vi "Auto_Routine_QuickAuto.vi"(8 "error in (no error)":errorcluster, 9 "Distance(Back)":dbl, 10 "Game Piece":T1, 11 "Position":T2=enum."Middle") -> (0 "error out":errorcluster)   [LabVIEW 2023]
uses:
  Arm/ArmPositionPreset.ctl
  Arm/ArmGamePiecePreset.ctl
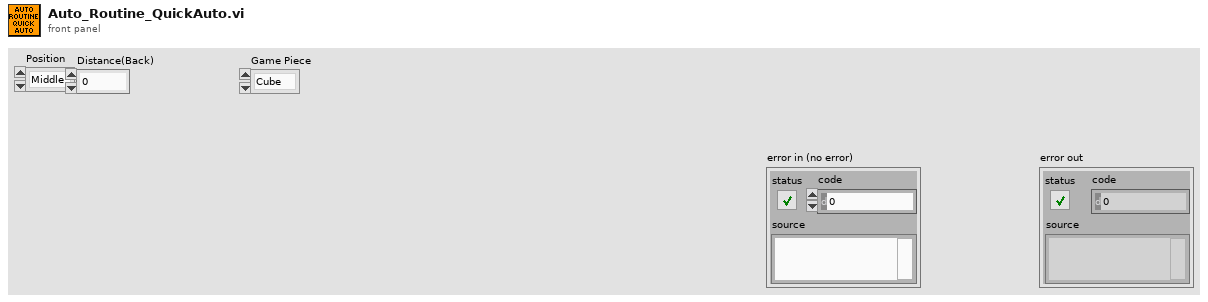
[diagram p1: front panel]
types:
  T1 = typedef "ArmGamePiecePreset.ctl" = enum16{"Cube", "Cone"}
  T2 = typedef "ArmPositionPreset.ctl" = enum16{"Upper", "Lower", "Middle", "Home", "Shelf", "Floor", "HalfFloor", "HalfHome"}
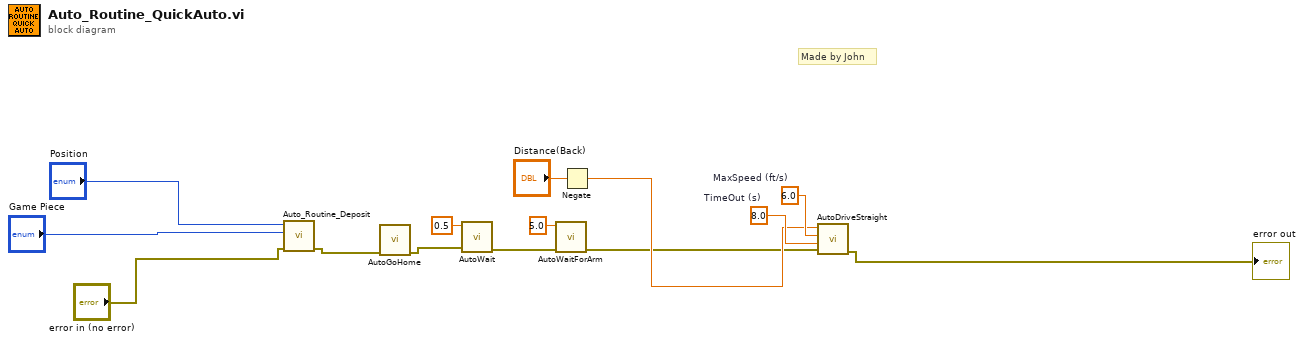
[diagram p0: block diagram]
diagram:
  w13 = 8.0  # TimeOut (s)
  w14 = 6.0  # MaxSpeed (ft/s)
  # "Made by John"
  n1 = call "Auto_Routine_Deposit.vi"("error in (no error)"="error in (no error)", "Game Piece"="Game Piece", "Position"="Position") -> ("error out"=w2:errorcluster)  [unwired: 8 in]
  n2 = call "AutoGoHome.vi"("error in (no error)"=w2) -> ("error out"=w3:errorcluster)  [unwired: 10 in]
  n3 = call "AutoWait.vi"("error in (no error)"=w3, "TimeOut (s)"=0.5) -> ("error out"=w5:errorcluster)  [unwired: 9 in]
  n4 = call "AutoWaitForArm.vi"("error in (no error)"=w5, "TimeOut (s)"=5.0) -> ("error out"=w1:errorcluster)  [unwired: 9 in]
  n5 = Negate(x="Distance(Back)") -> (-x=w8:dbl)
  n6 = call "AutoDriveStraight.vi"("error in (no error)"=w1, "TimeOut (s)"=w13, "MaxSpeed (ft/s)"=w14, "Dist (ft)"=w8) -> ("error out"=→"error out":errorcluster)  [unwired: 7 in]
